vi "testCreateConfigFilePath.vi"(8 "error in (no error)":errorcluster) -> (0 "error out":errorcluster)   [LabVIEW 2018]
doc: "Test the createConfigFilePath.vi"
uses:
  <vilib>/addons/_JKI Toolkits/Caraya/classes/Assert/Assert True.vi
  <vilib>/addons/_JKI Toolkits/Caraya/classes/Assert/Assert Equal Value_Variant.vi
  <vilib>/addons/_JKI Toolkits/Caraya/classes/Test/Test.lvclass
  <vilib>/addons/_JKI Toolkits/Caraya/classes/Assert/Assert.lvclass
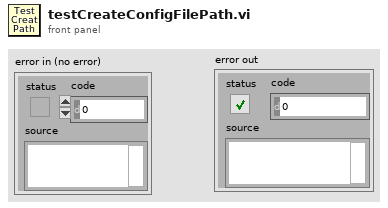
[diagram p1: front panel]
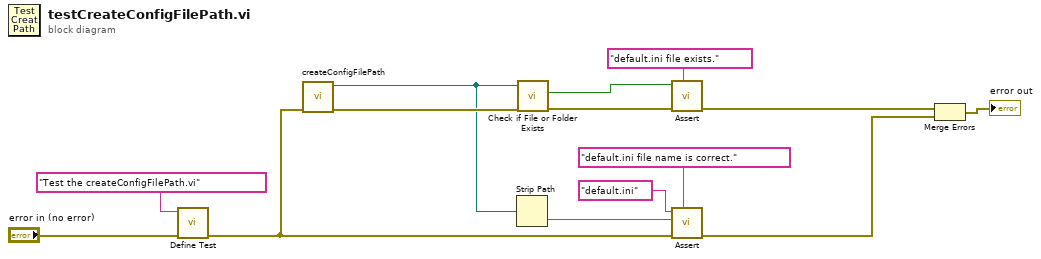
[diagram p0: block diagram]
diagram:
  n1 = call <vilib>:"Define Test.vi"("error in (no error)"="error in (no error)", "Label (VI Title)"="Test the createConfigFilePath.vi") -> ("error out"=w4:errorcluster)  [unwired: 9 in]
  n2 = call "createConfigFilePath.vi"("error in (no error)"=w4) -> ("error out"=w12:errorcluster, "ConfigFilePath"=w8:path)  [unwired: 9 in]
  n3 = Strip Path(path=w8) -> (name=w5:string)  [unwired: 1 out]
  n4 = call <vilib>:"Check if File or Folder Exists.vi"("error in (no error)"=w12, "path"=w8) -> ("error out"=w9:errorcluster, "file or folder exists?"=w11:bool)  [unwired: 7 in, 1 out]
  n5 = call-poly <vilib>:"Assert.vi"("Label"="default.ini file exists.", "error in (no error)"=w9, "True?"=w11) -> ("error out"=w3:errorcluster)  [unwired: 8 in]
  n6 = call-poly <vilib>:"Assert.vi"("Label"="default.ini file name is correct.", "error in (no error)"=w4, "Y"=w5, "X"="default.ini" ("Label")) -> ("error out"=w2:errorcluster)  [unwired: 7 in]
  n7 = Merge Errors(w3, w2) -> (→"error out":errorcluster)
